vi "Write Gantry Controller.vi"(8 "error in (no error)":errorcluster, 10 "Variant":variant, 11 "Gantry in":refnum<class "Gantry.lvclass">) -> (0 "error out":errorcluster, 3 "Gantry out":refnum<class "Gantry.lvclass">)   [LabVIEW 2024, in "Gantry.lvclass"]
uses:
  Gantry.lvclass
  Gantry.lvclass/Gantry.ctl
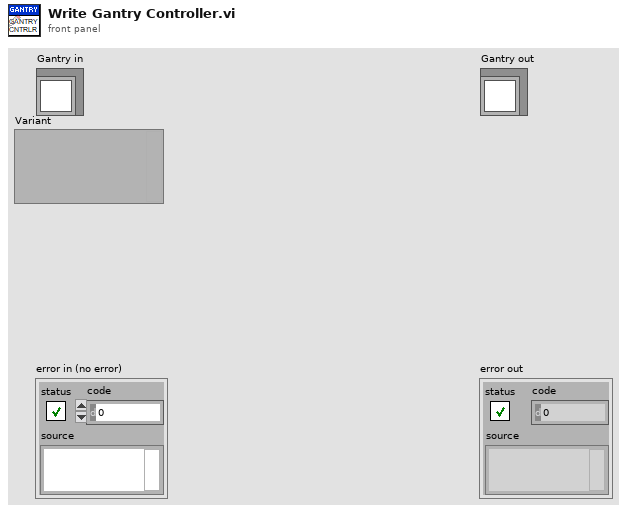
[diagram p1: front panel]
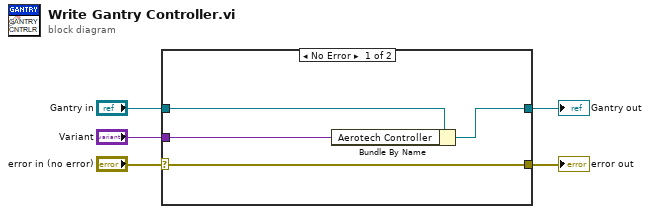
[diagram p0: block diagram]
diagram:
  n1 = case shown="No Error" "error in (no error)" {
    selector: "error in (no error)" -> [w9 w11]
    tunnel: [w9 w11] -> w4
    tunnel: [w6 w10] -> w2
    tunnel: "Gantry in" -> [w8 w10]
    tunnel: "Variant" -> [w7 _]
    frame No Error {
      n2 = Bundle By Name(cluster=w8, "Aerotech Controller"=w7) -> (w6:refnum<class "Gantry.lvclass">)
    }
    frame Error {
    }
  }
  "error out" <- w4
  "Gantry out" <- w2
